vi "Publish Scan Progress.vi"(8 "error in (no error)":errorcluster, 11 "Model in":refnum<class "Model.lvclass">) -> (0 "error out":errorcluster, 3 "Model out":refnum<class "Model.lvclass">)   [LabVIEW 2016, in "Model.lvclass"]
uses:
  Model.lvclass
  Typedefs/ScanProgress.ctl
  Typedefs/ActuatorData.ctl
  Model.lvclass/Model.ctl
  User Events/User Events.lvclass/User Events.ctl
  User Events/User Events.lvclass
  Typedefs/HPMT_Typedefs.lvlib
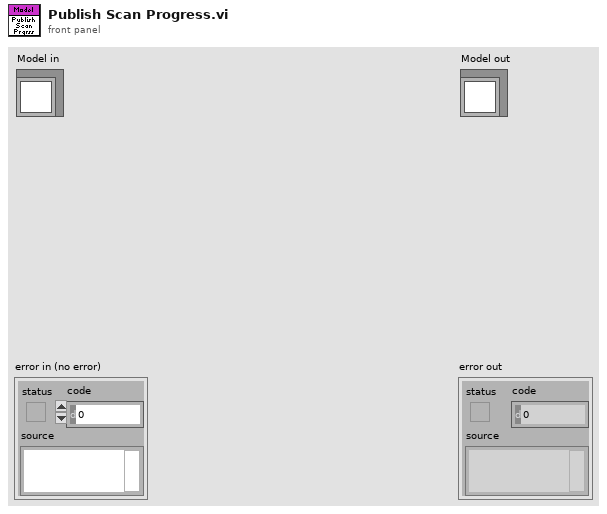
[diagram p1: front panel]
types:
  T1 = typedef "HPMT_Typedefs.lvlib/ScanProgress.ctl" = cluster{"Actuator Data":T2}
  T2 = typedef "HPMT_Typedefs.lvlib/ActuatorData.ctl" = cluster{"Timestamp":dbl, "Force":dbl, "Encoder Value":i32, "Displacement Sensor 1":dbl, "Displacement Sensor 2":dbl}
  T3 = typedef "HPMT_Typedefs.lvlib/Publish Data Events.ctl" = cluster{"State":refnum<user-event>, "ErrorCode":refnum<user-event>, "Scan Progress":refnum<user-event>, "All Test Status":refnum<user-event>, "ActuatorData":refnum<user-event>}
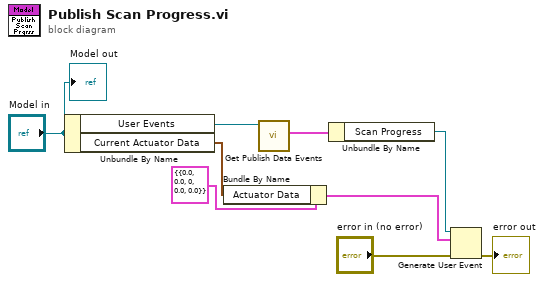
[diagram p0: block diagram]
diagram:
  n1 = Unbundle By Name("Model in") -> ("User Events"=w2:refnum<class "User Events.lvclass">, "Current Actuator Data"=w1:T2)
  n2 = Bundle By Name(cluster=T1 {"Actuator Data"={"Timestamp"=0.0, "Force"=0.0, "Encoder Value"=0, "Displacement Sensor 1"=0.0, "Displacement Sensor 2"=0.0}} ("event data"), "Actuator Data"=w1) -> (w4:T1)
  n3 = call "Get Publish Data Events.vi"("UserEvents in"=w2) -> ("Publish Data Events"=w8:T3)  [unwired: 9 in, 1 out]
  n4 = Unbundle By Name(w8) -> ("Scan Progress"=w9:refnum<user-event>)
  n5 = Generate User Event(user event=w9, event data cluster=w4, error in="error in (no error)") -> (error out=→"error out":errorcluster)  [unwired: 1 in, 1 out]
  "Model out" <- "Model in"
